vi "SENS_CORR_COLL_GUID_ACQ.vi"(0 "VISA IN":refnum<visa-resource-name>, 5 "error in":errorcluster, 7 "Channel":i32, 11 "Standerd":i32) -> (14 "VISA Out":refnum<visa-resource-name>, 19 "error out":errorcluster)   [LabVIEW 2018, in "PNA-X.lvlib"]
doc: "SENSe:CORRection:COLLect:GUIDed:ACQuire <std>\n(Write-only) Initiates the measurement of the specified calibration standard. Executing this command with an unnecessary standard has no affect.\n\nThe measured data is stored and used for subsequent calculations of error correction coefficients. All standards must be measured before a calibration can be completed. Any measurement can be repeated until the SENS:CORR:COLL:GUID:SAVE command is executed.\n\nQuery the user prompt description using SENS:CORR:COLL:GUID:DESC? \n\nQuery the required calibration steps using SENS:CORR:COLL:GUID:STEP?\n \nParameters\n \n \n<cnum>\n Any existing channel number. If unspecified, value is set to 1\n \n<std>\n Choose from:STAN1, STAN2, STAN3, through STAN40\n \nExamples\n SENS:CORR:COLL:GUID:ACQ STAN1\nsense:correction:collect:guided:acquire stan1\n \nQuery Syntax\n Not Applicable\n \nDefault\n Not Applicable"
uses:
  PNA-X.lvlib
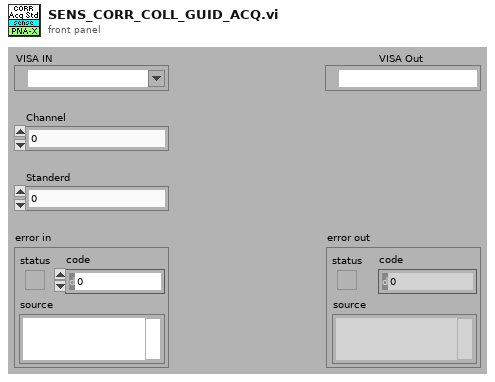
[diagram p1: front panel]
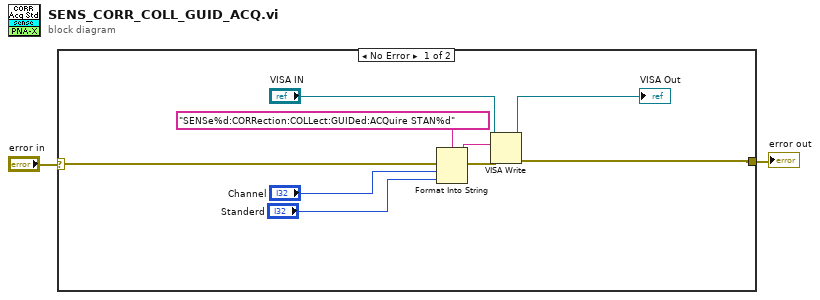
[diagram p0: block diagram]
diagram:
  n1 = case shown="No Error" "error in" {
    selector: "error in" -> [w11 w12]
    tunnel: [w6 w12] -> w1
    frame No Error {
      n2 = Format Into String(format string="SENSe%d:CORRection:COLLect:GUIDed:ACQuire STAN%d" ("Cmdline"), error in=w11, "Channel", "Standerd") -> (resulting string=w9:string, error out=w10:errorcluster)  [unwired: 1 in]
      n3 = VISA Write(VISA resource name="VISA IN", write buffer=w9, error in (no error)=w10) -> (VISA resource name out=→"VISA Out":refnum<visa-resource-name>, error out=w6:errorcluster)  [unwired: 1 out]
    }
    frame Error {
    }
  }
  "error out" <- w1
